vi "Query Reference Frequency Lock State.vi"(8 "error in (no error)":errorcluster, 11 "VISA resource name":refnum<visa-resource-name>) -> (0 "error out":errorcluster, 2 "Lock State":bool, 3 "VISA resource name out":refnum<visa-resource-name>)   [LabVIEW 2020, in "Rohde&Schwarz CMXP Base.lvlib"]
doc: "Queries whether the reference frequency is locked or not.\n\nAttribute:\nRSCMXPBASE_ATTR_REFERENCE_FREQUENCY_STATE\n\nRemote-control command:\nSENSe:BASE:REFerence:FREQuency:LOCKed?"
uses:
  <instrlib>/Rohde&Schwarz CMXP Base/Rohde&Schwarz CMXP Base.lvlib
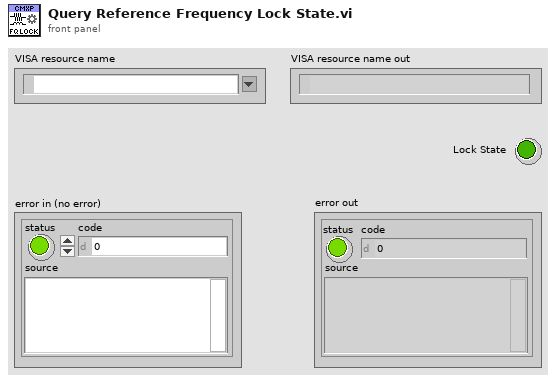
[diagram p1: front panel]
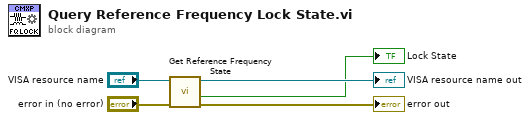
[diagram p0: block diagram]
diagram:
  n1 = call "Get Reference Frequency State"("error in (no error)"="error in (no error)", "instrument handle"="VISA resource name") -> ("error out"=→"error out":errorcluster, "Reference Frequency State"=→"Lock State":bool, "instrument handle out"=→"VISA resource name out":refnum<visa-resource-name>)  [unwired: 7 in]
